vi "Random.vi"() -> ()   [LabVIEW 2010]
uses:
  <vilib>/Utility/file.llb/Write To Spreadsheet File (DBL).vi
  <vilib>/Analysis/NI_AALBase.lvlib
panel:
  out "?":T1(graph)
  in  "Histogram Interval":dbl
  out "Graph of Random Numbers":dbl[](graph)
  in  "desired random number":dbl
  in  "Number random Numbers":dbl
  # "Histogram"
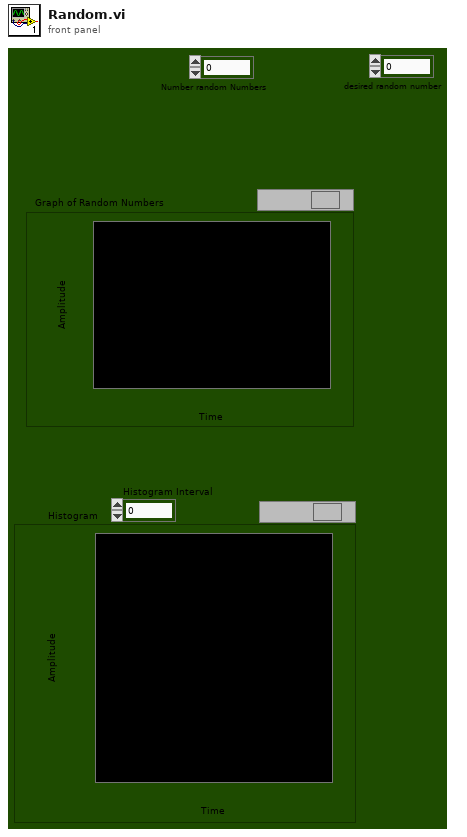
[diagram p1: front panel]
types:
  T1 = cluster{"X Values":dbl[], "Histogram: h(x)":i32[]}
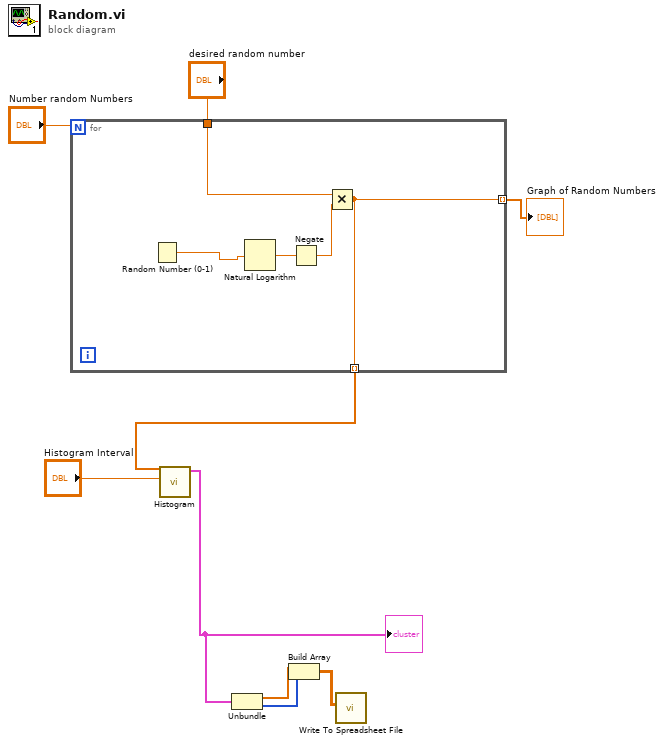
[diagram p0: block diagram]
diagram:
  n1 = for {
    N: "Number random Numbers" -> [_]
    tunnel: "desired random number" -> [w11]
    tunnel: [w10] -> w7 mode=indexing
    tunnel: [w10] -> w5 mode=indexing
    n2 = Random Number (0-1)() -> (number: 0 to 1=w14:dbl)
    n3 = Natural Logarithm(1:w14) -> (0:w13:dbl)
    n4 = Negate(x=w13) -> (-x=w12:dbl)
    n5 = Multiply(x=w11, y=w12) -> (x*y=w10:dbl)
  }
  "Graph of Random Numbers" <- w7
  n6 = call <vilib>:"Histogram.vi"("intervals"="Histogram Interval", "X"=w5) -> ("Histogram Graph"=w4:T1)  [unwired: 6 in, 3 out]
  "?" <- w4
  n7 = Unbundle(w4) -> ("X Values"=w3:dbl[], "Histogram: h(x)"=w2:i32[])
  n8 = Build Array(w3, w2) -> (w1:dbl[][])
  n9 = call-poly <vilib>:"Write To Spreadsheet File.vi"("2D data"=w1) -> ()  [unwired: 7 in, 1 out]
